vi "Ocean Optics 2000 4000 Acquire Continuous Waveform.vi"() -> ()   [LabVIEW 2013]
doc: "Demonstrates continuous waveform measurement. Spectrum is displayed in a waveform graph."
uses:
  <instrlib>/Ocean Optics 2000 4000/Ocean Optics 2000 4000.lvlib
panel:
  in  "Integration Time (6000)":u32=6000
  in  "Stop":bool
  out "Spectral Waveform":cluster{dbl[], dbl[]}(graph)
  in  "Enable Strobe (Disabled)":bool
  in  "VISA resource name":refnum<visa-resource-name>
  # "(c) 2009-2013 National Instruments.  ALL RIGHTS RESERVED."
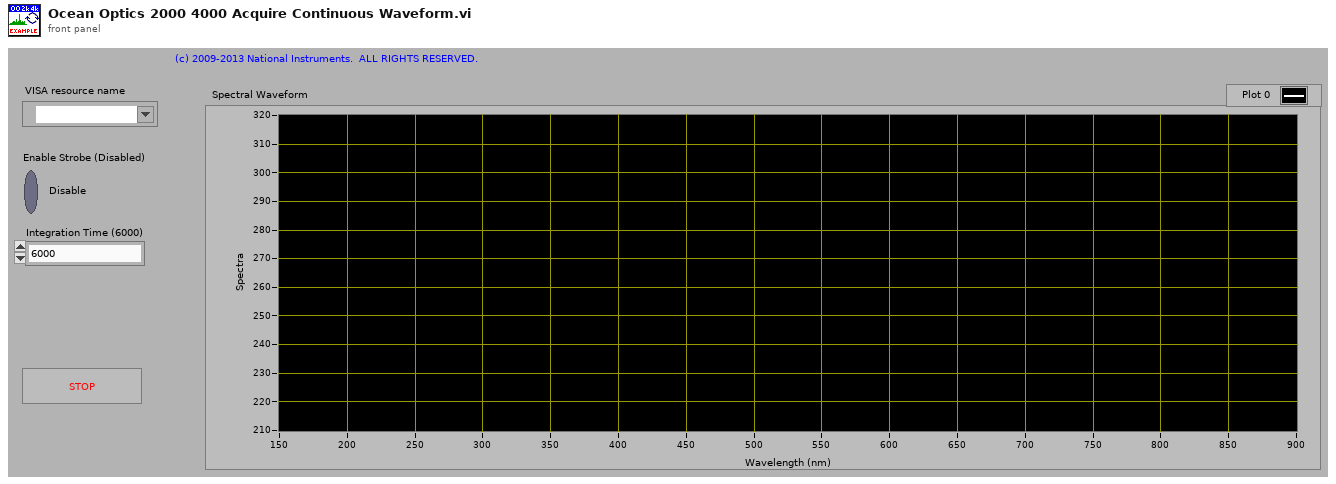
[diagram p1: front panel]
types:
  T1 = cluster{"Wavelength (nm)":dbl[], "Spectrum by Pixels":dbl[]}
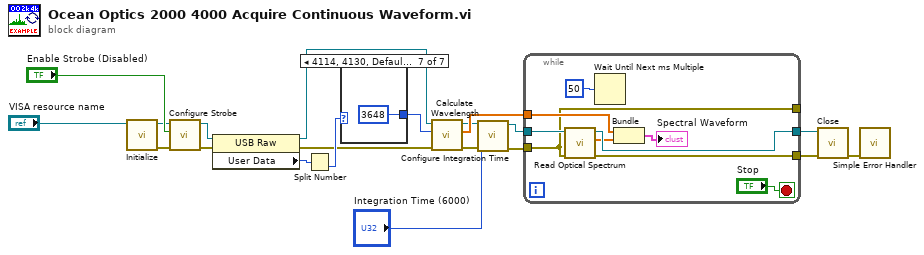
[diagram p0: block diagram]
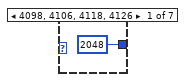
[diagram p2: hidden frame]
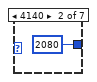
[diagram p3: hidden frame]
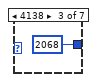
[diagram p4: hidden frame]
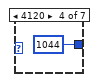
[diagram p5: hidden frame]
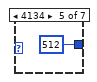
[diagram p6: hidden frame]
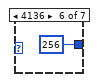
[diagram p7: hidden frame]
diagram:
  n1 = call <instrlib>:"Initialize.vi"("VISA resource name"="VISA resource name") -> ("error out"=w20:errorcluster, "VISA resource name out"=w6:refnum<visa-resource-name>)  [unwired: 9 in]
  n2 = call <instrlib>:"Configure Strobe.vi"("error in (no error)"=w20, "Enable Strobe (Disabled)"="Enable Strobe (Disabled)", "VISA resource name"=w6) -> ("error out"=w8:errorcluster, "VISA resource name out"=w9:refnum<visa-resource-name>)  [unwired: 7 in]
  n3 = property class="USB Raw"(reference=w9, error in=w8) -> (reference out=w11:refnum<visa-resource-name>, error out=w10:errorcluster, "User Data"=w14:u32)
  n4 = Split Number(x=w14) -> (lo(x)=w13:u16)  [unwired: 1 out]
  n5 = case shown="4114, 4130, Default" w13 {
    tunnel: [2048 ("Number of Pixels (3840)") 2080 ("Number of Pixels (3840)") 2068 ("Number of Pixels (3840)") 1044 ("Number of Pixels (3840)") 512 ("Number of Pixels (3840)") 256 ("Number of Pixels (3840)") 3648 ("Number of Pixels (3840)")] -> w12
    frame 4098, 4106, 4118, 4126 {
    }
    frame 4140 {
    }
    frame 4138 {
    }
    frame 4120 {
    }
    frame 4134 {
    }
    frame 4136 {
    }
    frame 4114, 4130, Default {
    }
  }
  n6 = call <instrlib>:"Calculate Wavelength.vi"("error in (no error)"=w10, "Number of Pixels (3648)"=w12, "VISA resource name"=w11) -> ("error out"=w4:errorcluster, "Wavelength (nm)"=w7:dbl[], "VISA resource name out"=w5:refnum<visa-resource-name>)  [unwired: 6 in]
  n7 = call <instrlib>:"Configure Integration Time.vi"("error in (no error)"=w4, "Integration Time (6000)"="Integration Time (6000)", "VISA resource name"=w5) -> ("error out"=w1:errorcluster, "VISA resource name out"=w2:refnum<visa-resource-name>)  [unwired: 7 in]
  n8 = while {
    tunnel: [w34] -> w18
    tunnel: [w33] -> w17
    tunnel: w7 -> [w32]
    tunnel: w2 -> [w30]
    tunnel: [w28] -> _
    tunnel: w1 -> [w28]
    stop <- "Stop" stop-if-true
    n9 = call <instrlib>:"Read Optical Spectrum.vi"("error in (no error)"=w28, "VISA resource name"=w30) -> ("error out"=w33:errorcluster, "Spectrum by Pixels"=w31:dbl[], "VISA resource name out"=w34:refnum<visa-resource-name>)  [unwired: 6 in, 1 out]
    n10 = Wait Until Next ms Multiple(millisecond multiple=u32 50) -> ()  [unwired: 1 out]
    n11 = Bundle("Wavelength (nm)"=w32, "Spectrum by Pixels"=w31) -> (→"Spectral Waveform":T1)  [unwired: 1 in]
  }
  n12 = call <instrlib>:"Close.vi"("error in (no error)"=w17, "VISA resource name"=w18) -> ("error out"=w16:errorcluster)  [unwired: 9 in]
  n13 = call <vilib>:"Simple Error Handler.vi"("error in (no error)"=w16) -> ()  [unwired: 4 in, 5 out]
